vi "Logic_Config_Capture_Duration.vi"(4 "error in (no error)":errorcluster, 6 "Capture Duration (s)":dbl=5.0 format="%#_13g", 7 "Session Ref In":T1) -> (0 "error out":errorcluster, 1 "Debug Status":string, 3 "Session Ref Out":T1)   [LabVIEW 2023]
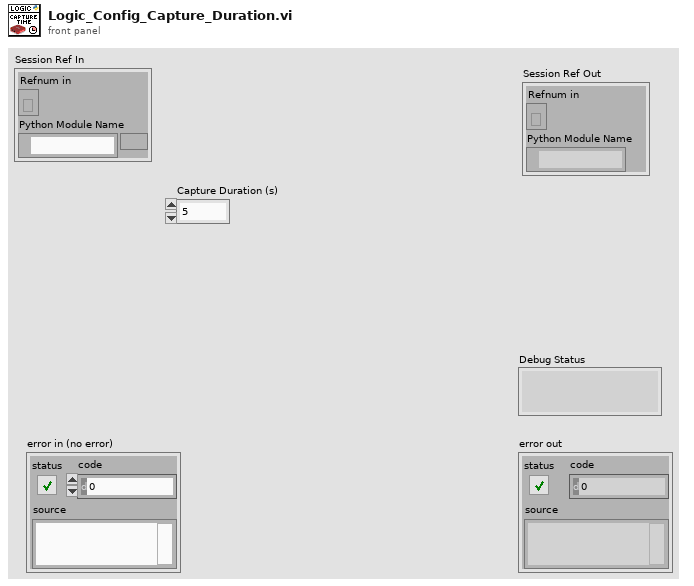
[diagram p1: front panel]
types:
  T1 = cluster{"Refnum in":refnum<k35>, "Python Module Name":path}
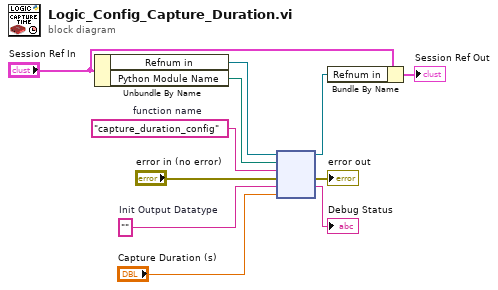
[diagram p0: block diagram]
diagram:
  w9 = "capture_duration_config"  # function name
  w8 = ""  # Init Output Datatype
  n1 = Unbundle By Name("Session Ref In") -> ("Refnum in"=w6:refnum<k35>, "Python Module Name"=w5:path)
  n2 = node(w6, w5, w9, "error in (no error)", w8, "Capture Duration (s)") -> (w3:refnum<k35>, →"error out":errorcluster, →"Debug Status":string)  [unwired: 1 in, 2 out]
  n3 = Bundle By Name(cluster="Session Ref In", "Refnum in"=w3) -> (→"Session Ref Out":T1)
